vi "PH_BeamlineController.set PA DP Target Attributes.vi"(0 "VI in":refnum<vi>, 2 "PA DP Target Index":i32, 3 "Changed PA DP Target Attributes":T1, 5 "error in (no error)":errorcluster) -> (14 "VI out":refnum<vi>, 19 "error out":errorcluster)   [LabVIEW 2014, in "PH_BeamlineController.lvlib"]
uses:
  PH_BeamlineController.lvlib
  PH_BeamlineController.PA DP Target Attributes.ctl
  PH_BeamlineController.PA DP Targets.ctl
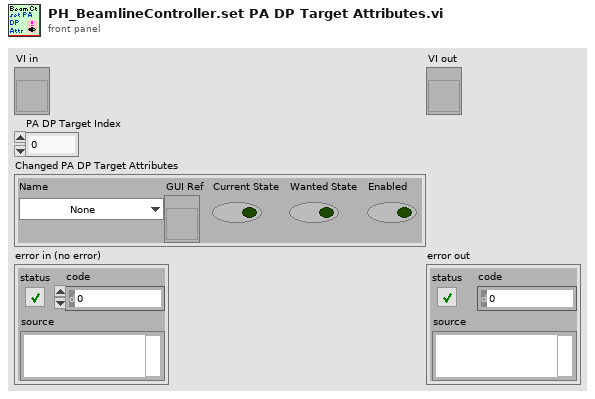
[diagram p1: front panel]
types:
  T1 = typedef "PH_BeamlineController.lvlib/PH_BeamlineController.PA DP Target Attributes.ctl" = cluster{"Name":T2, "GUI Ref":refnum<vi>, "Current State":bool, "Wanted State":bool, "Enabled":bool}
  T2 = typedef "PH_BeamlineController.lvlib/PH_BeamlineController.PA DP Targets.ctl" = enum16{"None", "Dump PA Delayed Beam", "Dump PA Undelayed Beam", "Dumps PA Delayed and Undelayed Beam"}
  T3 = typedef "PH_BeamlineController.lvlib/PH_BeamlineController.i attribute.ctl" = cluster{"Vacuum Exp LB":cluster{"Channel":string, "Limit [mbar]":dbl, "Pressure [mbar]":dbl, "GUI Ref":refnum<vi>}, "Sources":T4[], "PA DP Targets":T1[], "Path":cluster{"Source":T5, "PA DP Target":T2, "Target":T6}, "Targets":cluster{"Name":T6, "GUI Ref":refnum<vi>, "Current State":bool, "Wanted State":bool, "Enabled":bool}[], "Status Tags":cluster{"Name":string, "Status":T7}[], "special GUI Refs":T8}
  T4 = typedef "PH_BeamlineController.lvlib/PH_BeamlineController.Source Attributes.ctl" = cluster{"Name":T5, "GUI Ref":refnum<vi>, "Current State":bool, "Wanted State":bool}
  T5 = typedef "PH_BeamlineController.lvlib/PH_BeamlineController.Sources.ctl" = enum16{"None", "YLF", "fs-Frontend", "ns-Frontend", "YLF and ns-Frontend", "fs- and ns-Frontend"}
  T6 = typedef "PH_BeamlineController.lvlib/PH_BeamlineController.Targets.ctl" = enum16{"None", "PreAmp", "Dump Exp Laserlab", "Exp Laserlab", "Calorimeter", "Dump Exp Laserbay", "Exp Laserbay", "Dump Exp Z6", "Exp Z6"}
  T7 = typedef "PH_StatusHandler.lvlib/PH_StatusHandler.Status.ctl" = i16
  T8 = typedef "PH_BeamlineController.lvlib/PH_BeamlineController.special GUI Refs.ctl" = cluster{"PA-Backreflection-Meas":refnum<vi>, "fs_Synchrolock_Watch":refnum<vi>}
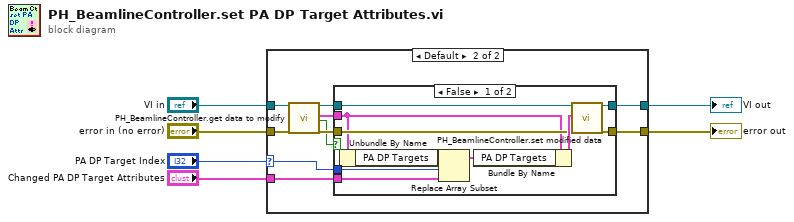
[diagram p0: block diagram]
diagram:
  n1 = case shown="Default" "PA DP Target Index" {
    selector: "PA DP Target Index" -> [_ w9]
    tunnel: "Changed PA DP Target Attributes" -> [_ w18]
    tunnel: "VI in" -> [w8 w17]
    tunnel: "error in (no error)" -> [w7 w16]
    tunnel: [w7 w15] -> w3
    tunnel: [w8 w14] -> w2
    frame -1 {
    }
    frame Default {
      n2 = call "PH_BeamlineController.get data to modify.vi"("i ref in"=w17, "error in (no error)"=w16) -> ("i ref out"=w13:refnum<vi>, "i attribute"=w11:T3, "timed out"=w10:bool, "error out"=w12:errorcluster)  [unwired: 14 in]
      n3 = case shown="False" w10 {
        tunnel: w13 -> [w25 w30]
        tunnel: [w28 w30] -> w14
        tunnel: w12 -> [w22 w29]
        tunnel: [w27 w29] -> w15
        tunnel: w11 -> [w21 _]
        tunnel: w18 -> [w19 _]
        tunnel: w9 -> [w24 _]
        frame False {
          n4 = Unbundle By Name(w21) -> ("PA DP Targets"=w20:T1[])
          n5 = Replace Array Subset(array=w20, new element=w19, index=w24) -> (w23:T1[])
          n6 = Bundle By Name(cluster=w21, "PA DP Targets"=w23) -> (w26:T3)
          n7 = call "PH_BeamlineController.set modified data.vi"("i ref in"=w25, "i attribute"=w26, "error in (no error)"=w22) -> ("i ref out"=w28:refnum<vi>, "error out"=w27:errorcluster)  [unwired: 15 in]
        }
        frame True {
        }
      }
    }
  }
  "error out" <- w3
  "VI out" <- w2
